vi "DriveS1P2.vi"   [LabVIEW 2016]
uses:
  <vilib>/Rock Robotics/WPI/SafetyOutput/WPI_SafetyOutputConfigMenu.ctl
  <vilib>/Rock Robotics/WPI/Utilities/WPI_GetSetVariantRefNum.vi
types:
  T1 = typedef "WPI_SafetyOutputConfigMenu.ctl" = enum16{"Enable", "Disable"}
  T2 = typedef "WPI_RobotDriveDevRef.ctl" = cluster{"DevStatus":errorcluster, "Motors[]":T3[], "Square Inputs":bool, "Max Output":dbl}
  T3 = typedef "WPI_MotorControlDeviceRef.ctl" = cluster{"DeviceStatus":errorcluster, "Type":T4, "PWM":cluster{"PWM Channel":T5, "DeadBand":T6}, "CAN":cluster{"Device Number":u8, "SetOutput VI Ref":variant, "GetOutput VI Ref":variant, "Enable VI Ref":variant, "Disable VI Ref":variant, "Data":variant}, "Invert":bool}
  T4 = typedef "WPI_MotorControlType.ctl" = enum16{"PWM", "CAN"}
  T5 = typedef "FPGA_DIOPWMChannel.ctl" = enum8{"PWM 0", "PWM 1", "PWM 2", "PWM 3", "PWM 4", "PWM 5", "PWM 6", "PWM 7", "PWM 8", "PWM 9", "PWM MXP 0", "PWM MXP 1", "PWM MXP 2", "PWM MXP 3", "PWM MXP 4", "PWM MXP 5", "PWM MXP 6", "PWM MXP 7", "PWM MXP 8", "PWM MXP 9", "Invalid"}
  T6 = typedef "WPI_PWMDeadband.ctl" = cluster{"Name":string, "maxPositivePwm":i32, "minPositivePwm":i32, "centerPwm":i32, "maxNegativePwm":i32, "minNegativePwm":i32, "angularRange":u16}
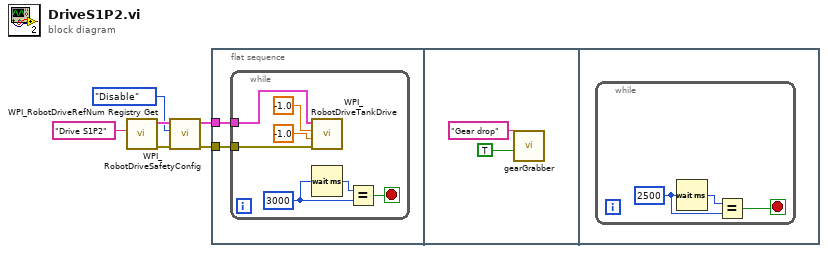
[diagram p0: block diagram]
diagram:
  n1 = call <vilib>:"WPI_RobotDriveRefNum Registry Get.vi"("refnum name"="Drive S1P2") -> ("error out"=w5:errorcluster, "RobotDriveDevRef"=w4:T2)  [unwired: 9 in]
  n2 = call <vilib>:"WPI_RobotDriveSafetyConfig.vi"("error in (no error)"=w5, "mode"=WPI_SafetyOutputConfigMenu."Disable", "RobotDriveDevRef"=w4) -> ("error out"=w1:errorcluster, "RobotDriveDevRef"=w2:T2)  [unwired: 7 in]
  n3 = flat-sequence {
    tunnel: w2 -> [w8]
    tunnel: w1 -> [w7]
    frame #0 {
      n4 = while {
        tunnel: w8 -> [w12]
        tunnel: w7 -> [w11]
        stop <- w13 stop-if-true
        w14 = u32 3000 ("milliseconds to wait")
        n5 = call <vilib>:"WPI_RobotDriveTankDrive.vi"("error in (no error)"=w11, "Right axis value"=-1.0, "Left axis value"=-1.0, "RobotDriveDevRef"=w12) -> ()  [unwired: 5 in, 3 out]
        n6 = Wait (ms)(milliseconds to wait=w14) -> (millisecond timer value=w15:u32)
        n7 = Equal?(x=w15, y=w14) -> (x = y?=w13:bool)
      }
    }
    frame #1 {
      n8 = call "gearGrabber.vi"("gearStatus"=TRUE, "gear"="Gear drop") -> ()  [unwired: 9 in, 1 out]
    }
    frame #2 {
      n9 = while {
        stop <- w18 stop-if-true
        w19 = u32 2500 ("milliseconds to wait")
        n10 = Wait (ms)(milliseconds to wait=w19) -> (millisecond timer value=w20:u32)
        n11 = Equal?(x=w20, y=w19) -> (x = y?=w18:bool)
      }
    }
  }
